vi "To Variant.vi"(0 "TTLDevice in":refnum<class "TTLWaterDelivery.lvclass">, 11 "error in (no error)":errorcluster) -> (4 "TTLDevice out":refnum<class "TTLWaterDelivery.lvclass">, 8 "Array":variant[](array[variant]), 15 "error out":errorcluster)   [LabVIEW 2020, in "TTLWaterDelivery.lvclass"]
uses:
  TTLWaterDelivery.lvclass
  TTLWaterDelivery.lvclass/TTLWaterDelivery.ctl
  Base Class/TTLControlledDevice.lvclass
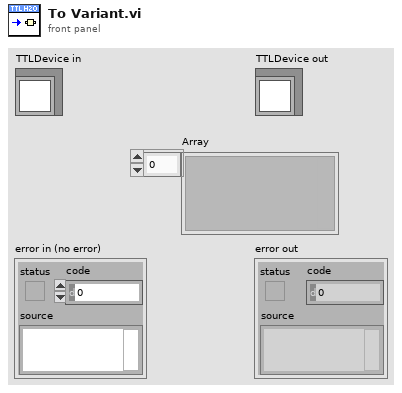
[diagram p1: front panel]
types:
  T1 = typedef "TTLWaterDelivery.lvclass/Serialized.ctl" = cluster{"uL/ms":dbl}
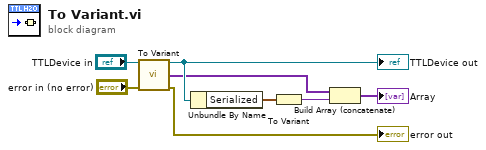
[diagram p0: block diagram]
diagram:
  n1 = call-parent "To Variant.vi"("TTLDevice in"="TTLDevice in", "error in (no error)"="error in (no error)") -> ("TTLDevice out"=w3:refnum<class "TTLWaterDelivery.lvclass">, "Array"=w2:variant[], "error out"=→"error out":errorcluster)  [unwired: 11 in]
  "TTLDevice out" <- w3
  n2 = Unbundle By Name(w3) -> ("Serialized"=w4:T1)
  n3 = To Variant(anything=w4) -> (Variant=w5:variant)
  n4 = Build Array (concatenate)(w2, w5) -> (→"Array":variant[])
